vi "De_Interleave.vi"(5 "Qm":dbl, 6 "C":dbl, 7 "rm_len":dbl[](array[numeric]), 8 "error in (no error)":errorcluster caption="错误输入（无错误）", 9 "EN_INTERWEAVER":dbl, 10 "deccbc_data":dbl[][](array[numeric]), 11 "appended path":path) -> (0 "error IO":errorcluster, 1 "deiwdata":dbl[][](array[numeric]))   [LabVIEW 2015]
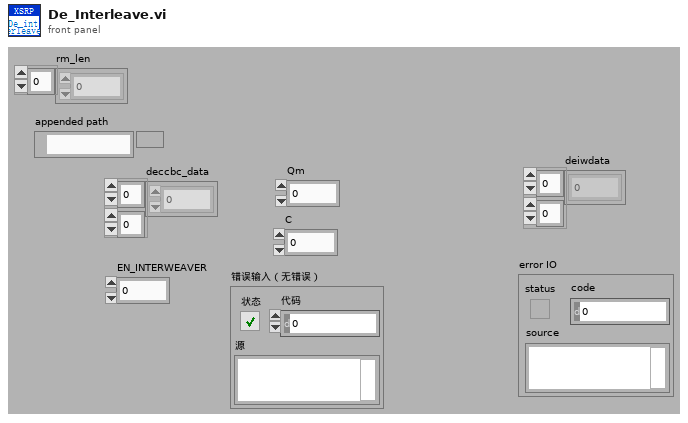
[diagram p1: front panel]
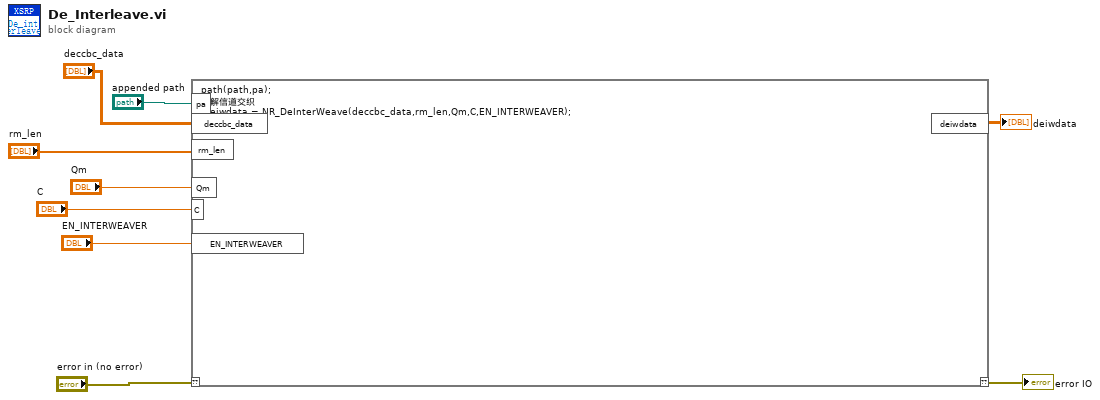
[diagram p0: block diagram]
diagram:
  n1 = script code="path(path,pa);\n%解信道交织\n deiwdata = NR_DeInterWeave(deccbc_data,rm_len,Qm,C,EN_INTERWEAVER);"("??"="error in (no error)", "pa"="appended path", "deccbc_data"="deccbc_data", "rm_len"="rm_len", "Qm"="Qm", "C"="C", "EN_INTERWEAVER"="EN_INTERWEAVER") -> ("??"=→"error IO":errorcluster, "deiwdata"=→"deiwdata":dbl[][])
